vi "Configure Arming.vi"(0 "VISA resource name":refnum<visa-resource-name>, 1 "Start Channel (0: A)":i32(ring) items=["A", "B", "E", "Off"], 2 "Start Slope (0: Positive)":i32(ring) items=["Positive", "Negative"], 5 "Bus Arming (T: On)":bool=TRUE, 7 "Start Arm Delay (20E-9)":dbl=2e-08, 9 "Arming Count (1)":i32=1, 11 "error in (no error)":errorcluster, 12 "Stop Channel (0: A)":i32(ring) items=["A", "B", "E", "Off"], 13 "Stop Slope (0: Positive)":i32(ring) items=["Positive", "Negative"]) -> (4 "VISA resource name out":refnum<visa-resource-name>, 15 "error out":errorcluster)   [LabVIEW 2019, in "Pendulum CNT90.lvlib"]
doc: "Configures start and stop arming and delay of start arming."
uses:
  Pendulum CNT90.lvlib
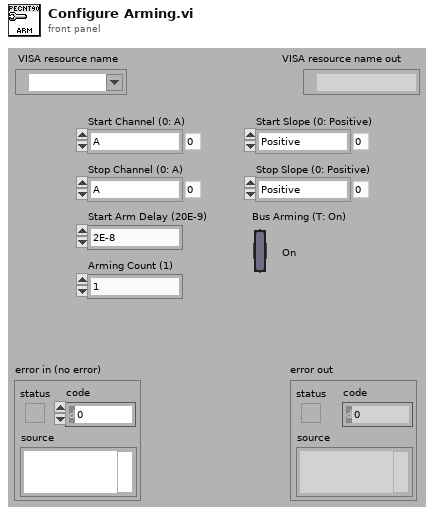
[diagram p1: front panel]
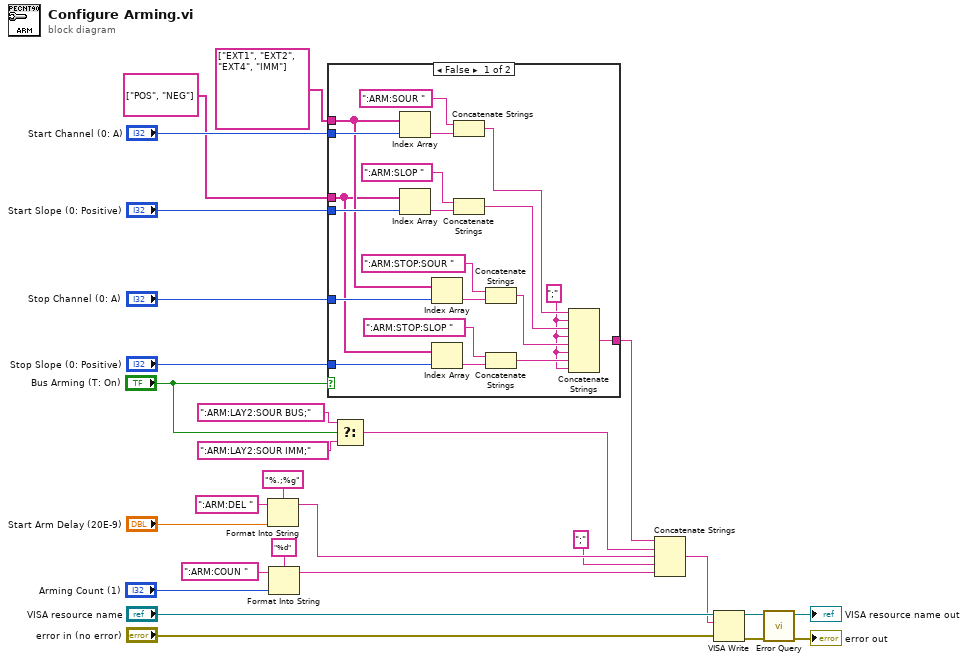
[diagram p0: block diagram]
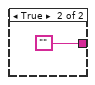
[diagram p2: hidden frame]
diagram:
  n1 = Format Into String(format string="%.;%g", initial string=":ARM:DEL ", "Start Arm Delay (20E-9)") -> (resulting string=w9:string)  [unwired: 1 in, 1 out]
  n2 = Format Into String(format string="%d", initial string=":ARM:COUN ", "Arming Count (1)") -> (resulting string=w8:string)  [unwired: 1 in, 1 out]
  n3 = case shown="False" "Bus Arming (T: On)" {
    tunnel: "Start Channel (0: A)" -> [w47 _]
    tunnel: "Start Slope (0: Positive)" -> [w43 _]
    tunnel: string[] ["EXT1", "EXT2", "EXT4", "IMM"] -> [w41 _]
    tunnel: "Stop Channel (0: A)" -> [w40 _]
    tunnel: string[] ["POS", "NEG"] -> [w39 _]
    tunnel: "Stop Slope (0: Positive)" -> [w38 _]
    tunnel: [w30 ""] -> w2
    frame False {
      w28 = ";" ("string")
      n4 = Index Array(array=w41, index=w47) -> (element=w45:string)
      n5 = Index Array(array=w39, index=w43) -> (element=w42:string)
      n6 = Index Array(array=w41, index=w40) -> (element=w37:string)
      n7 = Index Array(array=w39, index=w38) -> (element=w35:string)
      n8 = Concatenate Strings(":ARM:SOUR ", w45) -> (w29:string)
      n9 = Concatenate Strings(":ARM:SLOP ", w42) -> (w31:string)
      n10 = Concatenate Strings(":ARM:STOP:SOUR ", w37) -> (w33:string)
      n11 = Concatenate Strings(":ARM:STOP:SLOP ", w35) -> (w32:string)
      n12 = Concatenate Strings(w29, w28, w31, w28, w33, w28, w32, w28) -> (w30:string)
    }
    frame True {
    }
  }
  n13 = Select(t=":ARM:LAY2:SOUR BUS;", s="Bus Arming (T: On)", f=":ARM:LAY2:SOUR IMM;") -> (s? t:f=w4:string)
  n14 = Concatenate Strings(w2, w4, w9, ";" ("string"), w8) -> (w3:string)
  n15 = VISA Write(VISA resource name="VISA resource name", write buffer=w3, error in (no error)="error in (no error)") -> (VISA resource name out=w24:refnum<visa-resource-name>, error out=w21:errorcluster)  [unwired: 1 out]
  n16 = call "Error Query.vi"("error in (no error)"=w21, "VISA resource name"=w24) -> ("error out"=→"error out":errorcluster, "VISA resource name out"=→"VISA resource name out":refnum<visa-resource-name>)  [unwired: 6 in, 2 out]
